vi "PR Led Action.vi"(0 "Enable":bool) -> ()   [LabVIEW 2023, in "BS6006PRPLUS.lvlib"]
uses:
  BS6006PRPLUS.lvlib
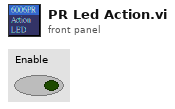
[diagram p1: front panel]
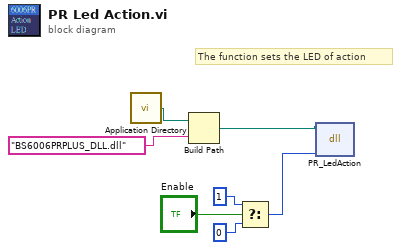
[diagram p0: block diagram]
diagram:
  # "The function sets the LED of action"
  n1 = call <vilib>:"Application Directory.vi"() -> ("Application Directory"=w7:path)
  n2 = Build Path(base path=w7, name or relative path="BS6006PRPLUS_DLL.dll") -> (appended path=w5:path)
  n3 = Select(t=u8 1, s="Enable", f=u8 0) -> (s? t:f=w1:u8)
  n4 = dll-call lib="C:/Users/BS/Desktop/LabVIEW 15/VIs/BS6006PRPLUS_DLL.dll" fn="PR_LedAction"(path in=w5, "Enable"=w1) -> ()  [unwired: 4 in, 2 out]
